vi "Part 2.vi"(11 "Input":string) -> (3 "Output":i64)   [LabVIEW 2021]
uses:
  <userlib>/_OpenG.lib/string/string.llb/Convert EOLs (String)__ogtk.vi
panel:
  out "Antenna positions":map{string, cluster{"Row":i32, "Col":i32}[]}(c390)
  out "Map":string[][](array[string])
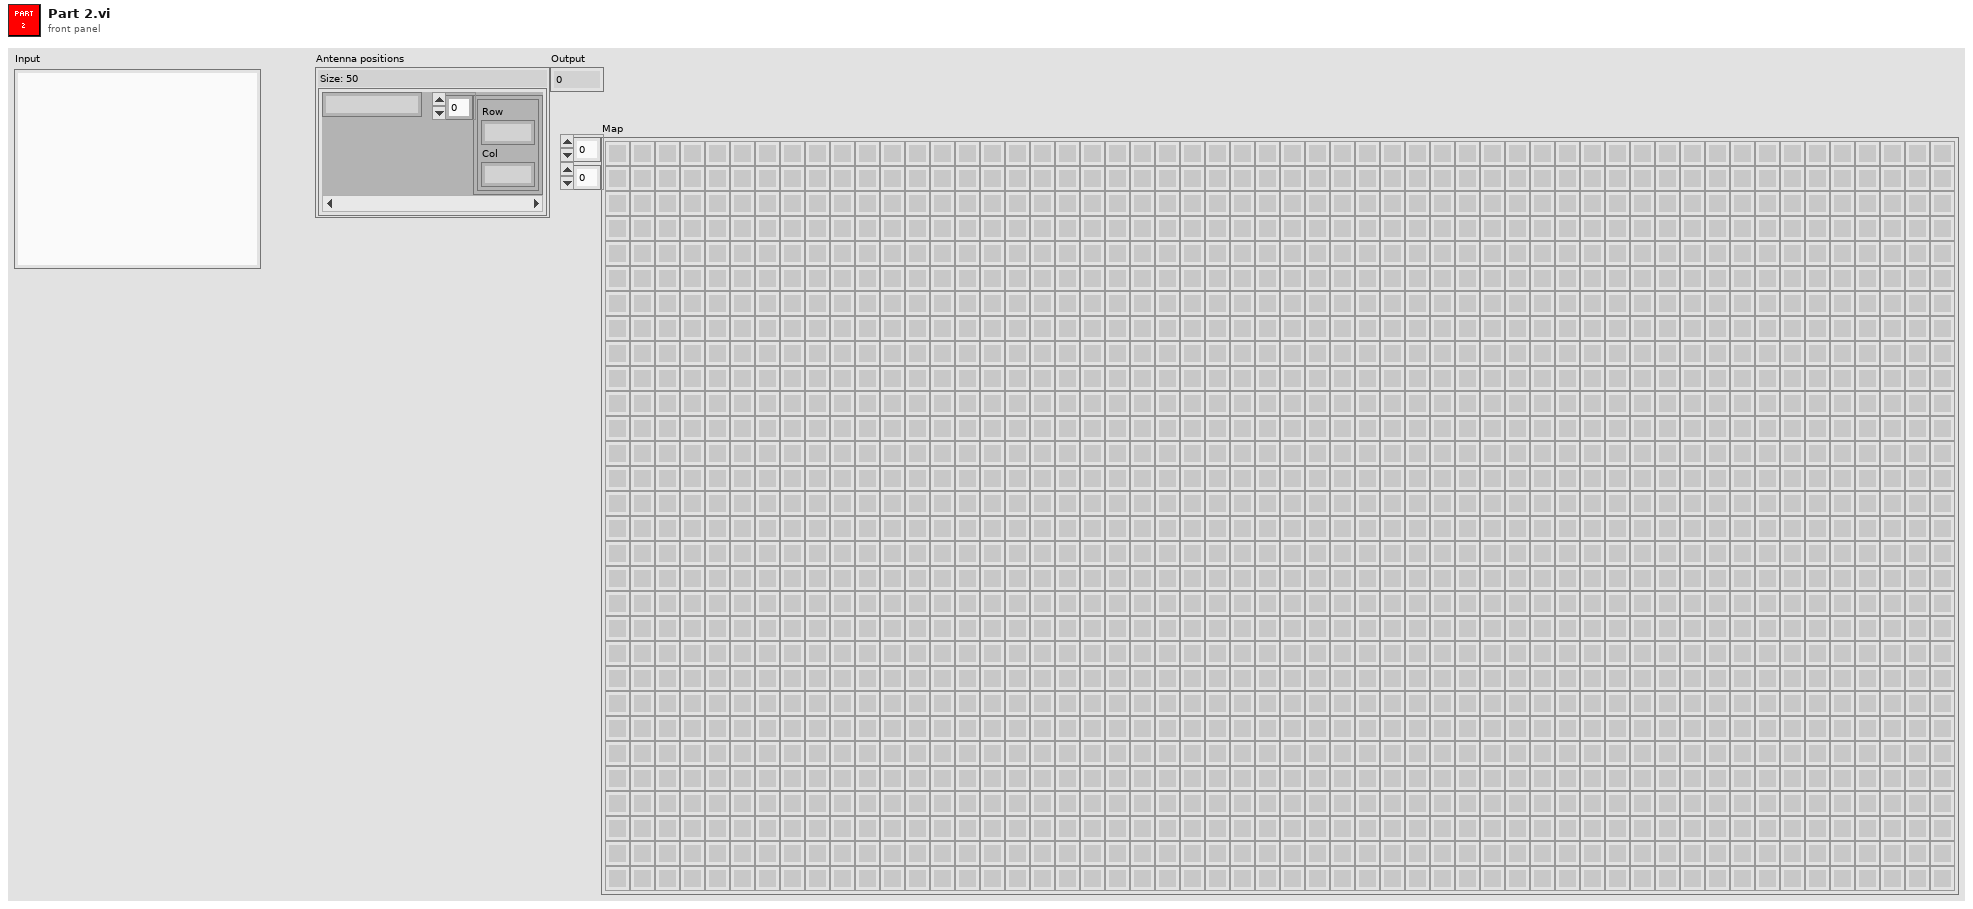
[diagram p1: front panel]
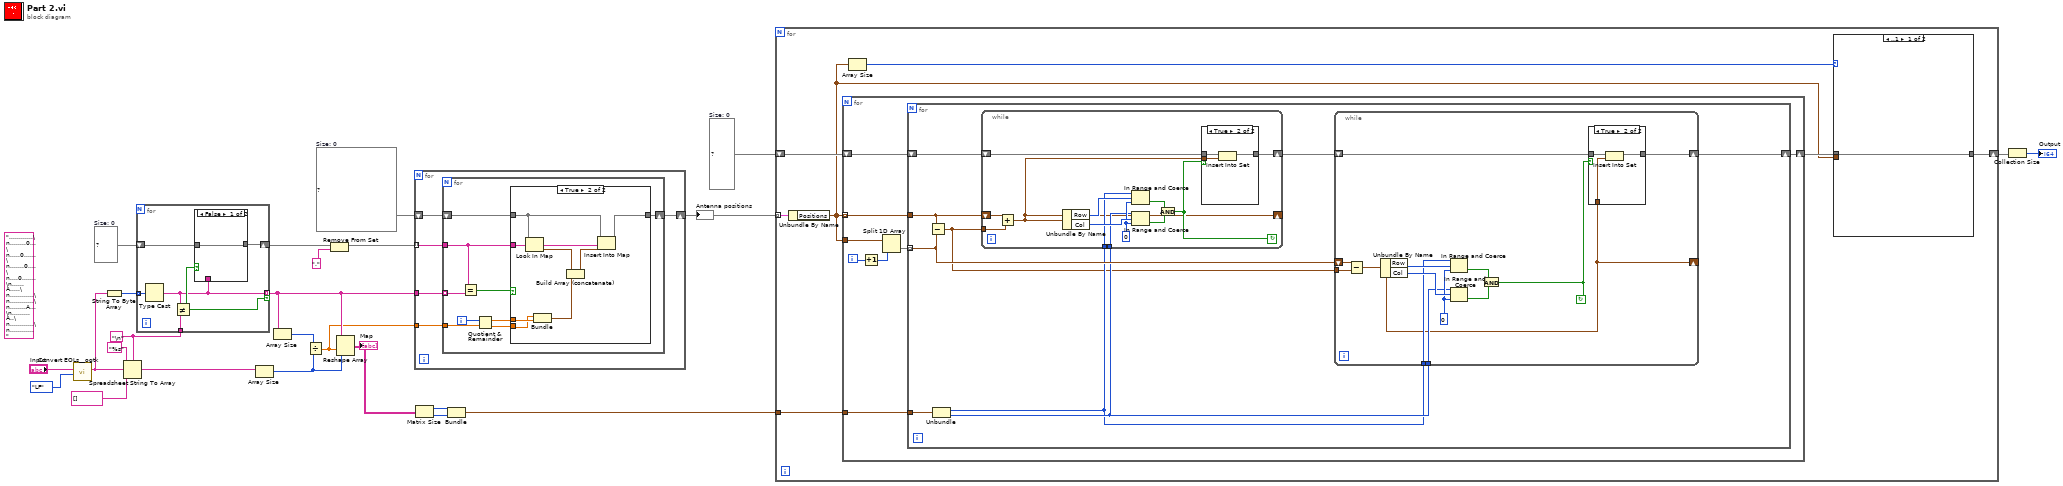
[diagram p0: block diagram]
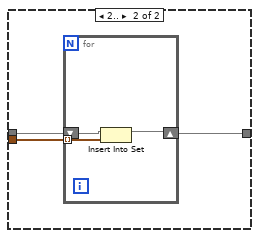
[diagram p2: hidden frame]
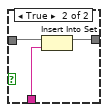
[diagram p6: hidden frame]
diagram:
  (unwired) "............\n........0...\n.....0......\n.......0....\n....0.......\n......A.....\n............\n............\n........A...\n.........A..\n............\n............"
  w8 = set{cluster{"Row":i32, "Col":i32}} {}  # Size: 0
  w14 = map{string, cluster{"Row":i32, "Col":i32}[]} {}  # Size: 0
  w16 = set{string} {}  # Size: 0
  w17 = "\n" ("delimiter (Tab)")
  n1 = call-poly <userlib>:"Convert EOLs__ogtk.vi"("Convert to:"=enum16{"CR", "LF", "CRLF"}."LF", "String in"="Input") -> ("String out"=w22:string)  [unwired: 9 in]
  n2 = String To Byte Array(string=w22) -> (unsigned byte array=w21:u8[])
  n3 = Spreadsheet String To Array(delimiter (Tab)=w17, format string="%s", spreadsheet string=w22, array type (2D Dbl)=string[] []) -> (array=w20:string[])
  n4 = for {
    tunnel: w21 -> [w31] mode=indexing
    tunnel: [w26] -> w13 mode=indexing if=w29
    tunnel: w17 -> [w30]
    shift-right: [w27] -> w15
    shift-left: w16 -> [w28]
    n5 = Type Cast(x=w31) -> (*(type *) &x=w26:string)  [unwired: 1 in]
    n6 = Not Equal?(x=w26, y=w30) -> (x != y?=w29:bool)
    n7 = case shown="False" w29 {
      tunnel: w28 -> [w32 w35]
      tunnel: [w32 w34] -> w27
      tunnel: w26 -> [_ w33]
      frame False {
      }
      frame True {
        n8 = Insert Into Set(10:w33, 11:w35) -> (3:w34:set{string})  [unwired: 1 out]
      }
    }
  }
  n9 = Array Size(array=w20) -> (size(s)=w19:i32)
  n10 = Array Size(array=w13) -> (size(s)=w18:i32)
  n11 = Divide(x=w18, y=w19) -> (x/y=w12:dbl)
  n12 = Remove From Set(10:".", 11:w15) -> (3:w11:set{string})  [unwired: 1 out]
  n13 = Reshape Array(w13, w12, w19) -> (w6:string[][])
  "Map" <- w6
  n14 = for {
    tunnel: w11 -> [w38] mode=indexing
    shift-right: [w36] -> w9
    shift-left: w14 -> [w37]
    tunnel: w13 -> [w40]
    tunnel: w12 -> [w39]
    n15 = for {
      tunnel: w40 -> [w47] mode=indexing
      tunnel: w39 -> [w48]
      tunnel: w38 -> [w43]
      shift-right: [w44] -> w36
      shift-left: w37 -> [w45]
      i -> [w49]
      n16 = Equal?(x=w43, y=w47) -> (x = y?=w46:bool)
      n17 = Quotient & Remainder(x=w49, y=w48) -> (x-y*floor(x/y)=w42:dbl, floor(x/y)=w41:dbl)
      n18 = case shown="True" w46 {
        tunnel: w45 -> [w50 w58]
        tunnel: [w50 w56] -> w44
        tunnel: w43 -> [_ w57]
        tunnel: w42 -> [_ w52]
        tunnel: w41 -> [_ w51]
        frame False {
        }
        frame True {
          n19 = Look In Map(map=w58, key=w57) -> (value=w55:cluster{"Row":i32, "Col":i32}[])  [unwired: 1 in, 1 out]
          n20 = Bundle(w51, w52) -> (w54:cluster{dbl, dbl})  [unwired: 1 in]
          n21 = Build Array (concatenate)(w55, w54) -> (w53:cluster{"Row":dbl, "Col":dbl}[])
          n22 = Insert Into Map(map in=w58, key=w57, value=w53) -> (map out=w56:map{string, cluster{"Row":i32, "Col":i32}[]})  [unwired: 2 out]
        }
      }
    }
  }
  "Antenna positions" <- w9
  n23 = Matrix Size(0:w6) -> (1:w4:i32, 2:w5:i32)
  n24 = Bundle("number of columns"=w4, "matrix"=w5) -> (w3:cluster{"number of columns":i32, "matrix":i32})  [unwired: 1 in]
  n25 = for {
    tunnel: w9 -> [w65] mode=indexing
    shift-right: [w60] -> w7
    shift-left: w8 -> [w64]
    tunnel: w3 -> [w63]
    n26 = Unbundle By Name(w65) -> ("Positions"=w59:cluster{"Row":i32, "Col":i32}[])
    n27 = for {
      tunnel: w59 -> [w77] mode=indexing
      tunnel: w59 -> [w80]
      shift-right: [w74] -> w61
      shift-left: w64 -> [w75]
      tunnel: w63 -> [w73]
      i -> [w79]
      n28 = Increment(x=w79) -> (x+1=w78:i32)
      n29 = Split 1D Array(array=w80, index=w78) -> (second subarray=w76:cluster{"Row":i32, "Col":i32}[])  [unwired: 1 out]
      n30 = for {
        tunnel: w77 -> [w81]
        tunnel: w76 -> [w89] mode=indexing
        shift-right: [w86] -> w74
        shift-left: w75 -> [w88]
        tunnel: w73 -> [w85]
        n31 = Subtract(x=w81, y=w89) -> (x-y=w82:cluster{"Row":i32, "Col":i32})
        n32 = Unbundle(w85) -> ("number of columns"=w83:i32, "matrix"=w84:i32)
        n33 = while {
          tunnel: w84 -> [w112]
          tunnel: w83 -> [w111]
          shift-right: [w118] -> w87
          shift-left: w88 -> [w119]
          tunnel: w82 -> [w109]
          shift-right: [w107] -> _
          shift-left: w81 -> [w110]
          stop <- w108 continue-if-true
          w113 = 0
          n34 = Add(x=w110, y=w109) -> (x+y=w107:cluster{"Row":i32, "Col":i32})
          n35 = Unbundle By Name(w107) -> ("Row"=w117:i32, "Col"=w116:i32)
          n36 = In Range and Coerce(upper limit=w111, x=w117, lower limit=w113) -> (In Range?=w114:bool)  [unwired: 1 out]
          n37 = In Range and Coerce(upper limit=w112, x=w116, lower limit=w113) -> (In Range?=w115:bool)  [unwired: 1 out]
          n38 = And(x=w114, y=w115) -> (x .and. y?=w108:bool)
          n39 = case shown="True" w108 {
            tunnel: w119 -> [w120 w123]
            tunnel: [w120 w122] -> w118
            tunnel: w107 -> [_ w121]
            frame False {
            }
            frame True {
              n40 = Insert Into Set(10:w121, 11:w123) -> (3:w122:set{cluster{"Row":i32, "Col":i32}})  [unwired: 1 out]
            }
          }
        }
        n41 = while {
          tunnel: w84 -> [w94]
          tunnel: w83 -> [w93]
          tunnel: w82 -> [w92]
          shift-right: [w100] -> w86
          shift-left: w87 -> [w101]
          shift-right: [w91] -> _
          shift-left: w89 -> [w102]
          stop <- w90 continue-if-true
          w97 = 0
          n42 = Subtract(x=w102, y=w92) -> (x-y=w91:cluster{"Row":i32, "Col":i32})
          n43 = Unbundle By Name(w91) -> ("Row"=w99:i32, "Col"=w98:i32)
          n44 = In Range and Coerce(upper limit=w93, x=w99, lower limit=w97) -> (In Range?=w95:bool)  [unwired: 1 out]
          n45 = In Range and Coerce(upper limit=w94, x=w98, lower limit=w97) -> (In Range?=w96:bool)  [unwired: 1 out]
          n46 = And(x=w95, y=w96) -> (x .and. y?=w90:bool)
          n47 = case shown="True" w90 {
            tunnel: w101 -> [w103 w106]
            tunnel: [w103 w105] -> w100
            tunnel: w91 -> [_ w104]
            frame False {
            }
            frame True {
              n48 = Insert Into Set(10:w104, 11:w106) -> (3:w105:set{cluster{"Row":i32, "Col":i32}})  [unwired: 1 out]
            }
          }
        }
      }
    }
    n49 = Array Size(array=w59) -> (size(s)=w62:i32)
    n50 = case shown="..1" w62 {
      tunnel: w61 -> [w66 w69]
      tunnel: [w66 w68] -> w60
      tunnel: w59 -> [_ w67]
      frame ..1 {
      }
      frame 2.. {
        n51 = for {
          shift-right: [w71] -> w68
          shift-left: w69 -> [w72]
          tunnel: w67 -> [w70] mode=indexing
          n52 = Insert Into Set(10:w70, 11:w72) -> (3:w71:set{cluster{"Row":i32, "Col":i32}})  [unwired: 1 out]
        }
      }
    }
  }
  n53 = Collection Size(1:w7) -> (0:→"Output":i32)
